vi "Cross Rough Terrain.vi"(11 "Event":T1) -> (3 "Next State":u16)   [LabVIEW 2016]
uses:
  Event.ctl
  State.ctl
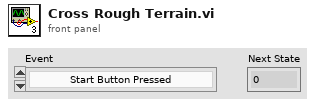
[diagram p1: front panel]
types:
  T1 = typedef "Event.ctl" = enum16{"Start Button Pressed", "Black & Yellow Tape Touched", "Black & Yellow Tape Passed", "Green Tape Crossed", "Red Tape Touched", "Rough Terrain Touched", "Black Tape Crossed", "Tape Edge Too Close", "Wall Too Close", "Rough Terrain Passed", "Ramp Passed", "Stop Button Pressed", "Recentered", "End Zone Wait Timed Out"}
  T2 = typedef "State.ctl" = enum16{"Wait", "Recenter", "Follow Wall", "Zig Zag", "Ramp", "Cross Rough Terrain", "Stagger Stop", "Obstacle Avoidance"}
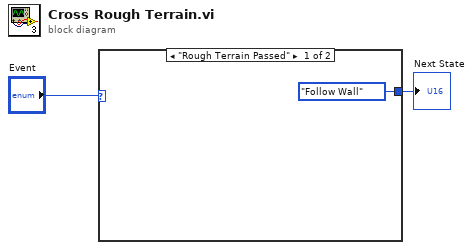
[diagram p0: block diagram]
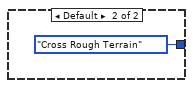
[diagram p2: hidden frame]
diagram:
  n1 = case shown="\"Rough Terrain Passed\"" "Event" {
    tunnel: [State."Follow Wall" ("State") State."Cross Rough Terrain" ("State")] -> w1
    frame "Rough Terrain Passed" {
    }
    frame Default {
    }
  }
  "Next State" <- w1
